vi "APC_CAD_derivative.vi"(1 "x (e.g., pcyl)":dbl[](array[numeric]), 2 "Encoder res. [CAD/sample]":dbl=0.1 format="%#_13g") -> (0 "dx/dCAD":dbl[](array[numeric]))   [LabVIEW 2020]
uses:
  <vilib>/Analysis/NI_AALPro.lvlib
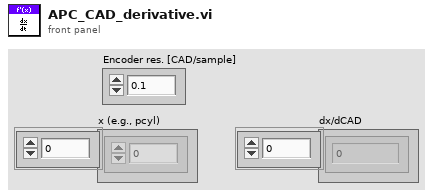
[diagram p1: front panel]
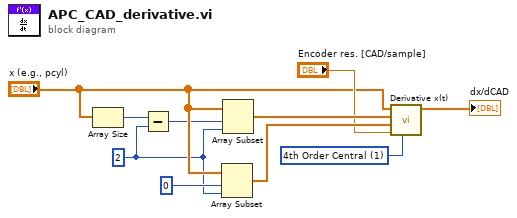
[diagram p0: block diagram]
diagram:
  w1 = 2 ("length")
  w10 = u16 1 items=["2nd Order Central", "4th Order Central", "Forward", "Backward"] ("method")
  n1 = Array Size(array="x (e.g., pcyl)") -> (size(s)=w3:i32)
  n2 = Subtract(x=w3, y=w1) -> (x-y=w2:i32)
  n3 = Array Subset(array="x (e.g., pcyl)", index=0, length=w1) -> (w7:dbl[])
  n4 = Array Subset(array="x (e.g., pcyl)", index=w2, length=w1) -> (w8:dbl[])
  n5 = call <vilib>:"Derivative x(t).vi"("method"=w10, "dt"="Encoder res. [CAD/sample]", "Final Condition"=w7, "Initial Condition"=w8, "X"="x (e.g., pcyl)") -> ("dX/dt"=→"dx/dCAD":dbl[])  [unwired: 5 in, 1 out]
